vi "get_PID.vi"(8 "error in (no error)":errorcluster, 11 "connection ID":refnum<k5>) -> (0 "error out":errorcluster, 2 "PID cluster":cluster{"P":dbl, "I":dbl, "D":dbl}, 3 "connection ID out":refnum<k5>)   [LabVIEW 2018]
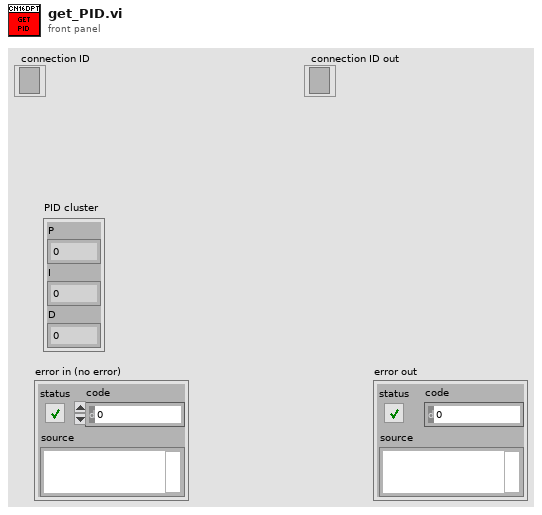
[diagram p1: front panel]
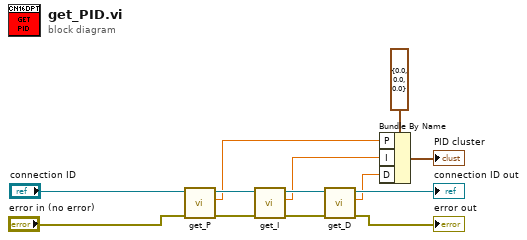
[diagram p0: block diagram]
diagram:
  n1 = call "get_P.vi"("error in (no error)"="error in (no error)", "connection ID"="connection ID") -> ("error out"=w10:errorcluster, "P"=w5:dbl, "connection ID out"=w13:refnum<k5>)  [unwired: 7 in]
  n2 = call "get_I.vi"("error in (no error)"=w10, "connection ID"=w13) -> ("error out"=w9:errorcluster, "I"=w4:dbl, "connection ID out"=w12:refnum<k5>)  [unwired: 7 in]
  n3 = call "get_D.vi"("error in (no error)"=w9, "connection ID"=w12) -> ("error out"=→"error out":errorcluster, "D"=w3:dbl, "connection ID out"=→"connection ID out":refnum<k5>)  [unwired: 7 in]
  n4 = Bundle By Name(cluster=cluster{"P":dbl, "I":dbl, "D":dbl} {"P"=0.0, "I"=0.0, "D"=0.0} ("PID cluster"), "P"=w5, "I"=w4, "D"=w3) -> (→"PID cluster":cluster{"P":dbl, "I":dbl, "D":dbl})
